vi "FF_AnkleTraj2.vi"(6 "Init":bool, 7 "dt":dbl=0.01 format="%0.2f", 8 "error in (no error)":errorcluster, 9 "AnkleVelocity":dbl[](array[numeric]), 10 "AnkleInGCS":dbl[](array[numeric]), 11 "Force Field Controller in":refnum<class "ForceField.lvclass">) -> (0 "error out":errorcluster, 1 "ClosePt":dbl[](array[numeric]), 2 "Force":dbl[](array[numeric]), 3 "Force Field Controller out":refnum<class "ForceField.lvclass">, 5 "ForceComp":dbl[](array[numeric]))   [LabVIEW 2015, in "ForceField.lvclass"]
uses:
  ForceField.lvclass
  ForceField.lvclass/ForceField.ctl
  <vilib>/ptbypt/NI_PtbyPt.lvlib
panel:
  in  "Xmin":dbl=0.1 format="%#_13g"
  out "ActiveTraj":dbl[][](array[numeric])
  in  "HalfWindow":i32=35
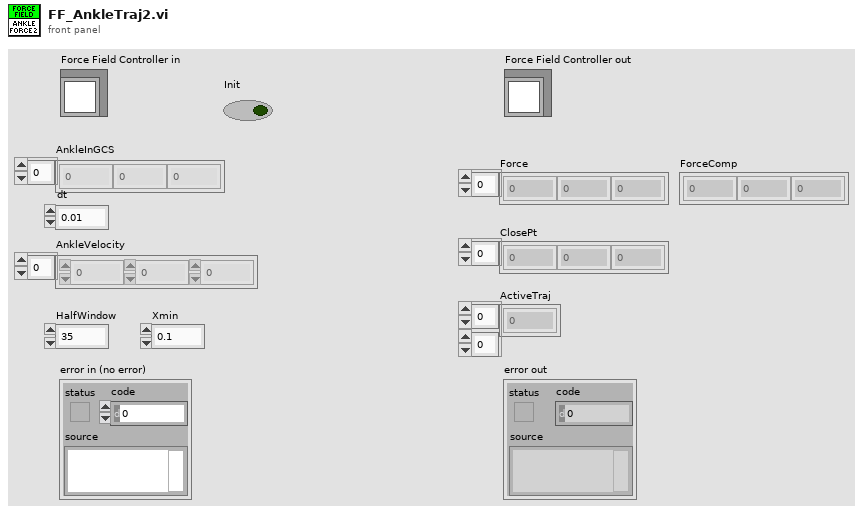
[diagram p1: front panel]
types:
  T1 = typedef "ForceField.lvclass/AnkleTrajPt.ctl" = cluster{"P1":dbl[], "P2":dbl[], "P1-P2":dbl[], "(P1-P2)^2":dbl}
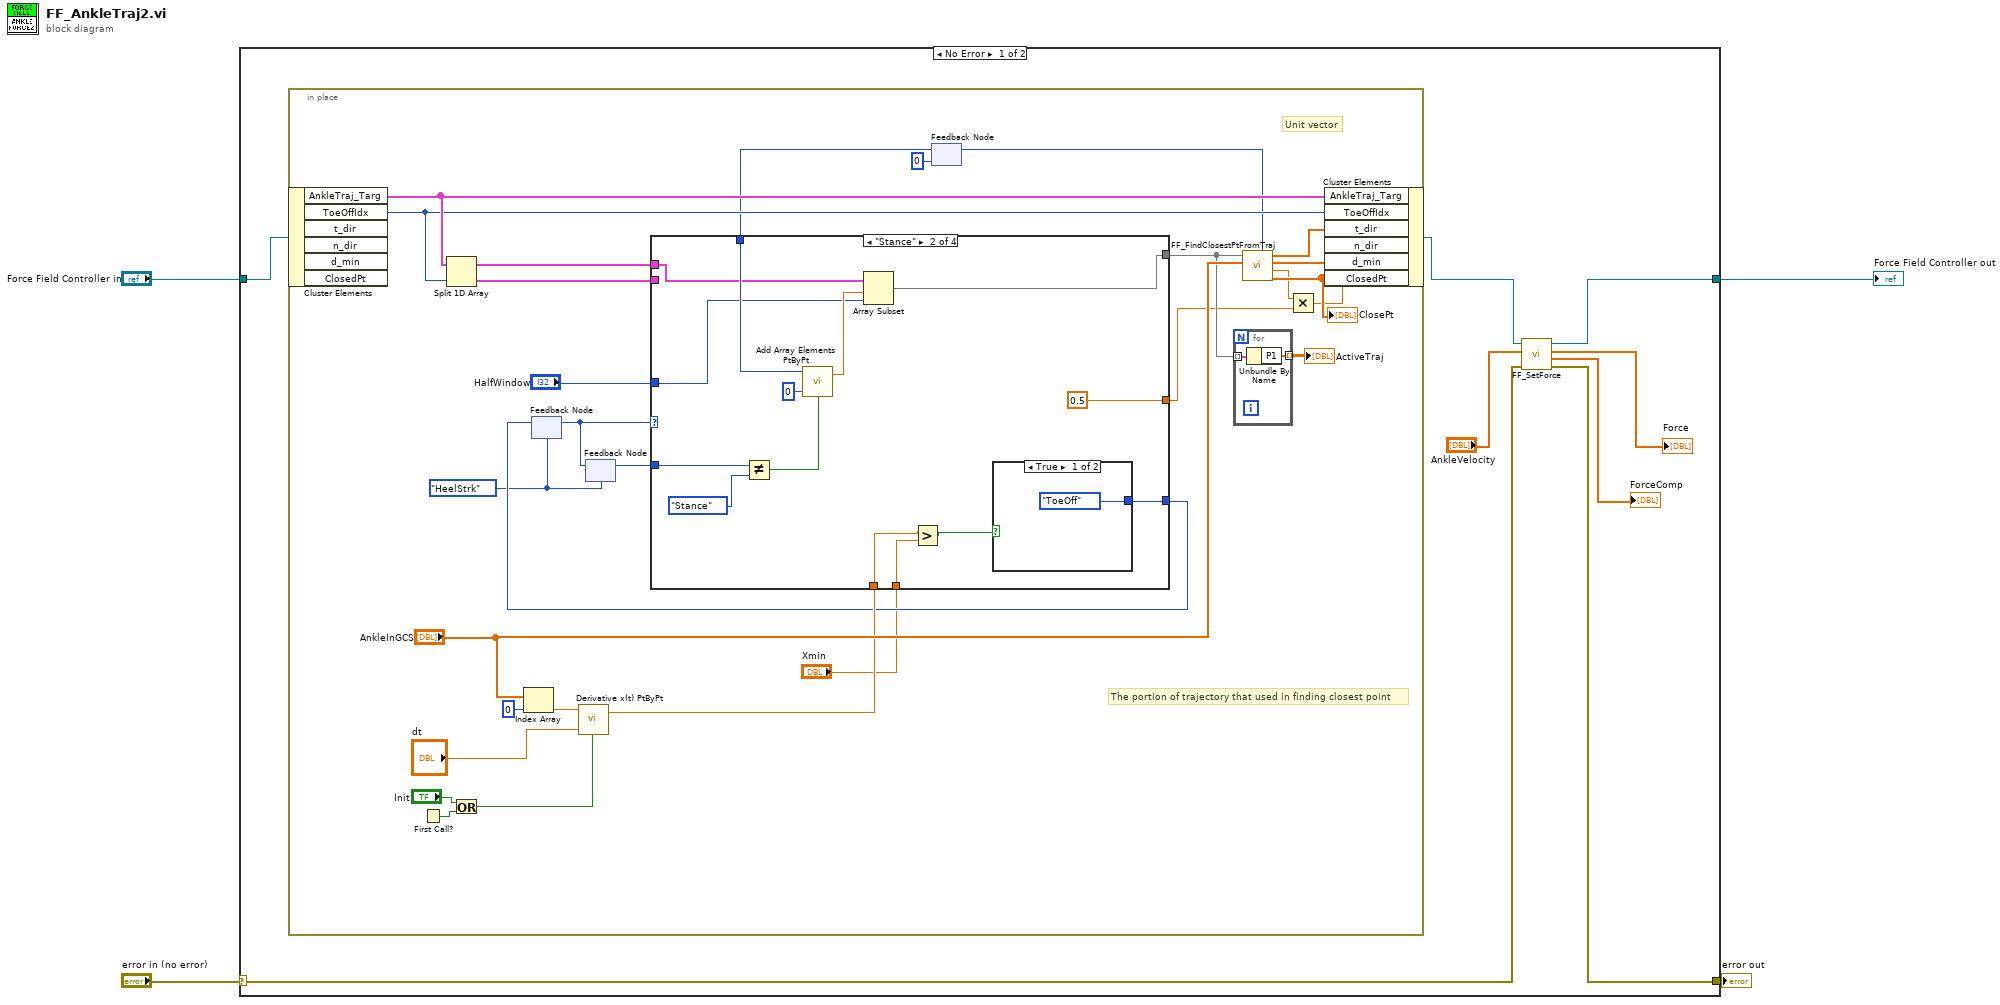
[diagram p0: block diagram]
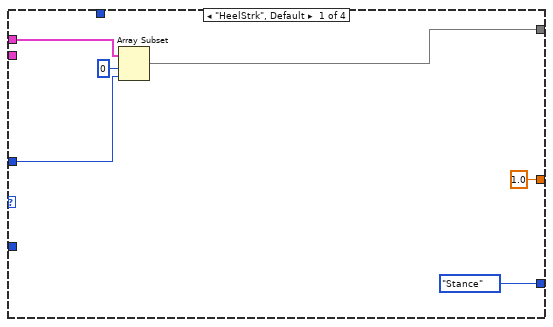
[diagram p2: hidden frame]
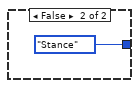
[diagram p3: hidden frame]
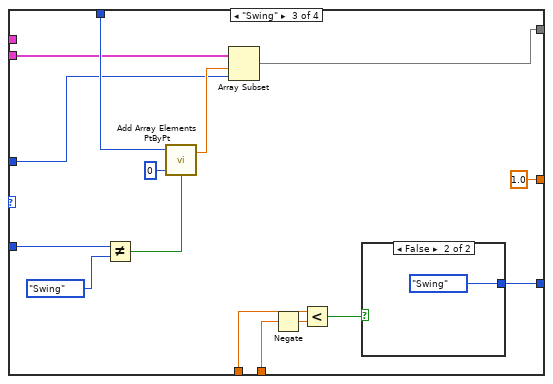
[diagram p4: hidden frame]
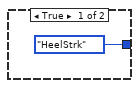
[diagram p5: hidden frame]
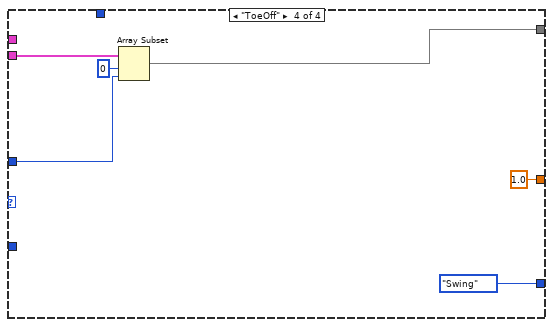
[diagram p6: hidden frame]
diagram:
  n1 = case shown="No Error" "error in (no error)" {
    selector: "error in (no error)" -> [w8 w90]
    tunnel: [w7 w90] -> w3
    tunnel: [w10 w89] -> w1
    tunnel: "Force Field Controller in" -> [w12 w89]
    frame No Error {
      n2 = in-place {
        w18 = enum16{"HeelStrk", "Stance", "ToeOff", "Swing"}."HeelStrk"
        # "The portion of trajectory that used in finding closest point"
        # "Unit vector"
        n3 = in-place-cluster #1(w12) -> ("AnkleTraj_Targ"=w30:T1[], "ToeOffIdx"=w29:i32)  [unwired: 4 out]
        n4 = First Call?() -> (First Call?: T/F=w41:bool)
        n5 = Split 1D Array(array=w30, index=w29) -> (first subarray=w28:T1[], second subarray=w27:T1[])
        n6 = Or(x="Init", y=w41) -> (x .or. y?=w32:bool)
        n7 = Index Array(array="AnkleInGCS", index=0) -> (element=w33:dbl)
        n8 = feedback #2(w18) -> (w19:enum16{"HeelStrk", "Stance", "ToeOff", "Swing"})
        n9 = call <vilib>:"Derivative x(t) PtByPt.vi"("initialize"=w32, "dt"="dt", "x"=w33) -> ("dx/dt"=w21:dbl)  [unwired: 1 in, 1 out]
        n10 = feedback #3(w18) -> (w17:enum16{"HeelStrk", "Stance", "ToeOff", "Swing"})
        n11 = feedback-in #3(w19) -> ()
        n12 = feedback #4(0 ("IndexOfClosePt")) -> (w25:i32)
        n13 = case shown="\"Stance\"" w19 {
          tunnel: w28 -> [w43 w51 _ _]
          tunnel: w27 -> [_ _ w68 w82]
          tunnel: "HalfWindow" -> [w45 w59 w76 w84]
          tunnel: [w47 w55 w72 w86] -> w22
          tunnel: [enum16{"HeelStrk", "Stance", "ToeOff", "Swing"}."Stance" w54 w70 enum16{"HeelStrk", "Stance", "ToeOff", "Swing"}."Swing"] -> w20
          tunnel: w25 -> [_ w61 w78 _]
          tunnel: w21 -> [_ w53 w69 _]
          tunnel: w17 -> [_ w50 w67 _]
          tunnel: [1.0 0.5 1.0 1.0] -> w15
          tunnel: "Xmin" -> [_ w48 w64 _]
          frame "HeelStrk", Default {
            n14 = Array Subset(array=w43, index=0, length=w45) -> (w47:T1[])
          }
          frame "Stance" {
            n15 = Not Equal?(x=w50, y=enum16{"HeelStrk", "Stance", "ToeOff", "Swing"}."Stance") -> (x != y?=w57:bool)
            n16 = call <vilib>:"Add Array Elements PtByPt.vi"("initialize"=w57, "sample length"=0, "input data point"=w61) -> ("sum"=w60:dbl)  [unwired: 1 in, 1 out]
            n17 = Array Subset(array=w51, index=w60, length=w59) -> (w55:T1[])
            n18 = Greater?(x=w53, y=w48) -> (0:w52:bool)
            n19 = case shown="True" w52 {
              tunnel: [enum16{"HeelStrk", "Stance", "ToeOff", "Swing"}."ToeOff" enum16{"HeelStrk", "Stance", "ToeOff", "Swing"}."Stance"] -> w54
              frame True {
              }
              frame False {
              }
            }
          }
          frame "Swing" {
            n20 = Not Equal?(x=w67, y=enum16{"HeelStrk", "Stance", "ToeOff", "Swing"}."Swing") -> (x != y?=w74:bool)
            n21 = call <vilib>:"Add Array Elements PtByPt.vi"("initialize"=w74, "sample length"=0, "input data point"=w78) -> ("sum"=w77:dbl)  [unwired: 1 in, 1 out]
            n22 = Array Subset(array=w68, index=w77, length=w76) -> (w72:T1[])
            n23 = Negate(x=w64) -> (-x=w65:dbl)
            n24 = Less?(x=w69, y=w65) -> (x < y?=w71:bool)
            n25 = case shown="False" w71 {
              tunnel: [enum16{"HeelStrk", "Stance", "ToeOff", "Swing"}."HeelStrk" enum16{"HeelStrk", "Stance", "ToeOff", "Swing"}."Swing"] -> w70
              frame True {
              }
              frame False {
              }
            }
          }
          frame "ToeOff" {
            n26 = Array Subset(array=w82, index=0, length=w84) -> (w86:T1[])
          }
        }
        n27 = feedback-in #2(w20) -> ()
        n28 = for {
          tunnel: [w88] -> w36 mode=indexing
          tunnel: w22 -> [w87] mode=indexing
          n29 = Unbundle By Name(w87) -> ("P1"=w88:dbl[])
        }
        "ActiveTraj" <- w36
        n30 = call "FF_FindClosestPtFromTraj.vi"("AnkleInGCS"="AnkleInGCS", "AnkleTraj"=w22) -> ("ClosestPt"=w39:dbl[], "DistanceToClosestPt"=w16:dbl, "NormalVectorToClosestPt"=w37:dbl[], "TangentVectorAtClosestPt"=w38:dbl[], "IndexOfClosePt"=w26:i32)  [unwired: 5 in]
        "ClosePt" <- w39
        n31 = feedback-in #4(w26) -> ()
        n32 = Multiply(x=w16, y=w15) -> (x*y=w14:dbl)
        n33 = in-place-cluster #1("AnkleTraj_Targ"=w30, "ToeOffIdx"=w29, "t_dir"=w38, "n_dir"=w37, "d_min"=w14, "ClosedPt"=w39) -> (w11:refnum<class "ForceField.lvclass">)
      }
      n34 = call "FF_SetForce.vi"("error in (no error)"=w8, "AnkleVelocity"="AnkleVelocity", "Force Field Controller in"=w11) -> ("error out"=w7:errorcluster, "ForceNTD"=→"ForceComp":dbl[], "ForceXYZ"=→"Force":dbl[], "Force Field Controller out"=w10:refnum<class "ForceField.lvclass">)  [unwired: 5 in]
    }
    frame Error {
    }
  }
  "error out" <- w3
  "Force Field Controller out" <- w1
